vi "Lidar Main V5.2.vi"() -> ()   [LabVIEW 2015]
uses:
  <vilib>/Utility/error.llb/Error Cluster From Error Code.vi
  <vilib>/rvi/errors/niLvFpgaAdjustHostInterfaceError.vi
  Program Files (x86)/National Instruments/LabVIEW 2015/Targets/NI/FPGA/StockFPGA_IntfPrivate/ScriptTemplates/StockFPGA_PlugInRead32.vi
  <vilib>/FPGAPlugInAG/PXIe-7972R/niLvFpga_Abort_PXIe-7972R.vi
  <vilib>/rvi/interface/nirviReadWriteControl/nirviReadWriteControl.xnode
  Controls/FpgaMasterRef Typedef.ctl
  FPGA Bitfiles/LidarMasterV5.1.4.lvbitx
  Controls/FpgaSlaveRef Typedef.ctl
  FPGA Bitfiles/LidarSlaveV5.1.4.lvbitx
  <vilib>/rvi/interface/nirviMethod/nirviMethod.xnode
  <vilib>/rvi/errors/niLvFpgaMergeErrorWithErrorCode.vi
  NiFpgaLv.dll
  <vilib>/FPGAPlugInAG/PXIe-7972R/niLvFpga_Read32_PXIe-7972R.vi
  <vilib>/rvi/interface/nirviReadWriteControl/niFpgaRWControlAccessTimeoutTemplate.vi
  <vilib>/FPGAPlugInAG/PXIe-7972R/niLvFpga_ReadFifo_PXIe-7972R.vi
panel:
  out "RawData":u32[](array[numeric])
  out "error out 2":errorcluster
  out "# elements in queue 2":i32
  out "error out":errorcluster
  in  "SendUDP":bool
  in  "Set VGA Const.":bool
  in  "VGA Val":i16
  out "String":string
  in  "Delay&Close":bool
  in  "SaveToFile":bool
  in  "StartAcq":u16=26 caption="Start Acquisition"
  in  "ActiveSensDeb":u8 caption="Active Sensor"
  in  "SensScanDeb":bool caption="Sensor Scan"
  in  "Active VCSL":u16
  in  "LedScanDebEn":bool=TRUE caption="VCSL Scan"
  in  "Fill VGA":bool
  in  "VGA data":i16[](array[numeric])=[15000, 15000, 15000, 15000, 15000, 15000, 15000, 15000, 15000, 15000, 15000, 15000, 15000, 15000, 15000, 15000, 15000, 15000, 15000, 15000, 15000, 15000, 15000, 15000, 15000, 15000, 15000, 15000, 15000, 15000, 15000, 15000, 15000, 15000, 15000, 15000, 15000, 15000, 15000, 15000, 15000, 15000, 15000, 15000, 15000, 15000, 15000, 15000, 15000, 15000, 15000, 15000, 15000, 15000, 15000, 15000, 15000, 15000, 15000, 15000, 15000, 15000, 15000, 15000, 15000, 15000, 15000, 15000, 15000, 15000, 15000, 15000, 15000, 15000, 15000, 15000, 15000, 15000, 15000, 15000, 15000, 15000, 15000, 15000, 15000, 15000, 15000, 15000, 15000, 15000, 15000, 15000, 15000, 15000, 15000, 15000, 15000, 15000, 15000, 15000]
  in  "PulseEnd":u16=25
  in  "StartPulse":u16=20
  in  "StartES":u16=38
  in  "StopES":u16=44
  in  "SamplingEnable":bool caption="Acquire Frames no Graph"
  in  "AcqMode":bool=TRUE caption="Acq. Mode (T=Raw)"
  in  "SingleFrame":bool caption="Acquire Single Frame"
  out "Samples Amount":i32
  in  "Go":bool caption="Acquire Frames With Graph"
  out "File Error":errorcluster
  in  "CloseFile":bool
  in  "OpenFile":bool
  out "Elements Remaining":u32
  out "Data":i16[][](graph)
  in  "stop":bool
  out "FPGA Error":errorcluster
  # "Acquisition Control"
  # "Timing Control"
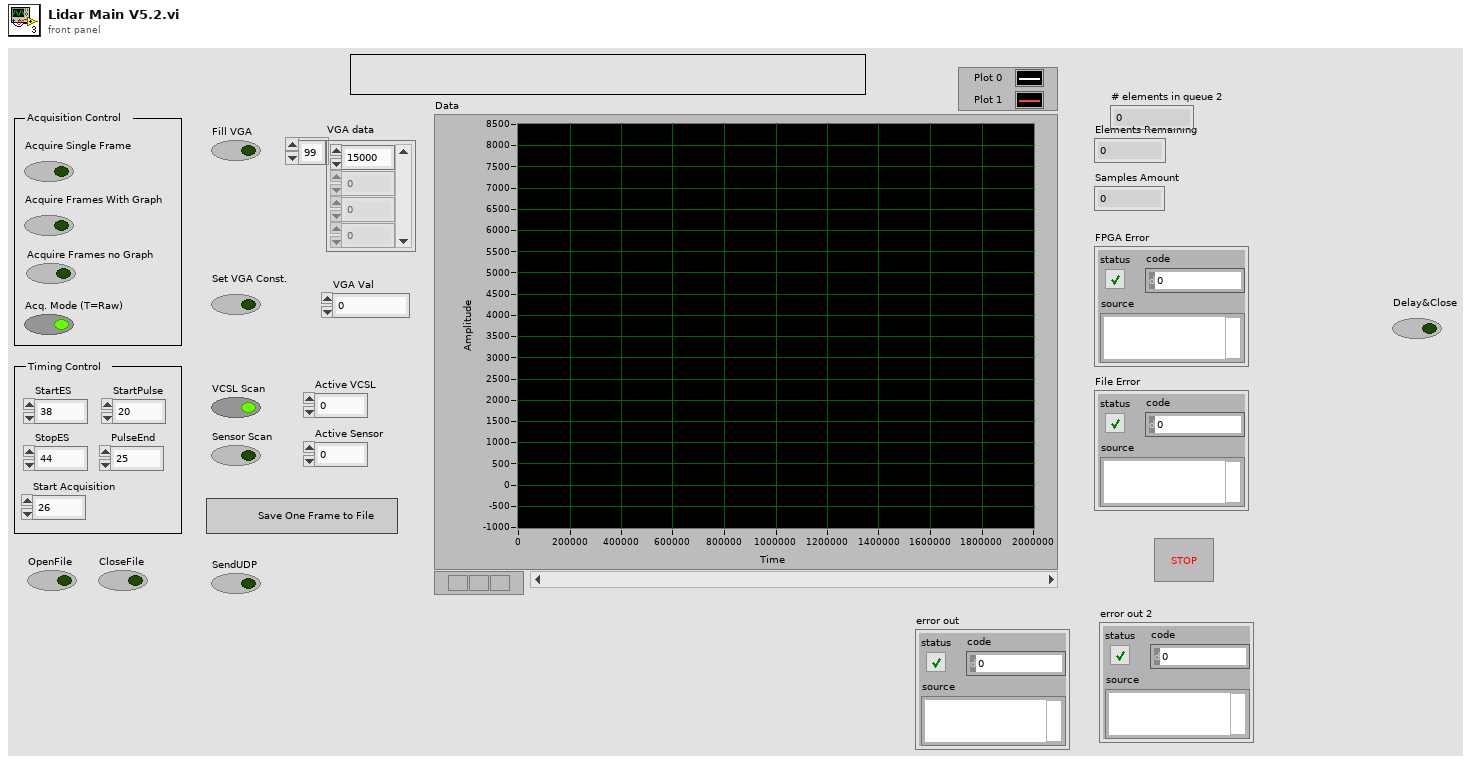
[diagram p1: front panel]
types:
  T1 = enum8{"Internal Clock PLL Off", "Internal Clock PLL On (CLK IN)", "External Clock (CLK IN)", "Internal Clock PLL On (IoModSyncClock)", "Extrernal Clock (IoModSyncClk)"}
  T2 = enum8{"Internal Clock PLL Off", "Internal Clock PLL On (CLK_IN)", "External Clock (CLK_IN)", "Internal Clock PLL On (IoModSyncClk)", "External Clock (IoModSyncClk)"}
  T3 = typedef "FpgaSlaveRef Typedef.ctl" = refnum<k20>
  T4 = typedef "FpgaMasterRef Typedef.ctl" = refnum<k20>
  T5 = enum16{"open", "replace", "create", "open or create", "replace or create", "replace or create with confirmation"}
  T6 = enum16{"big-endian, network order", "native, host order", "little-endian"}
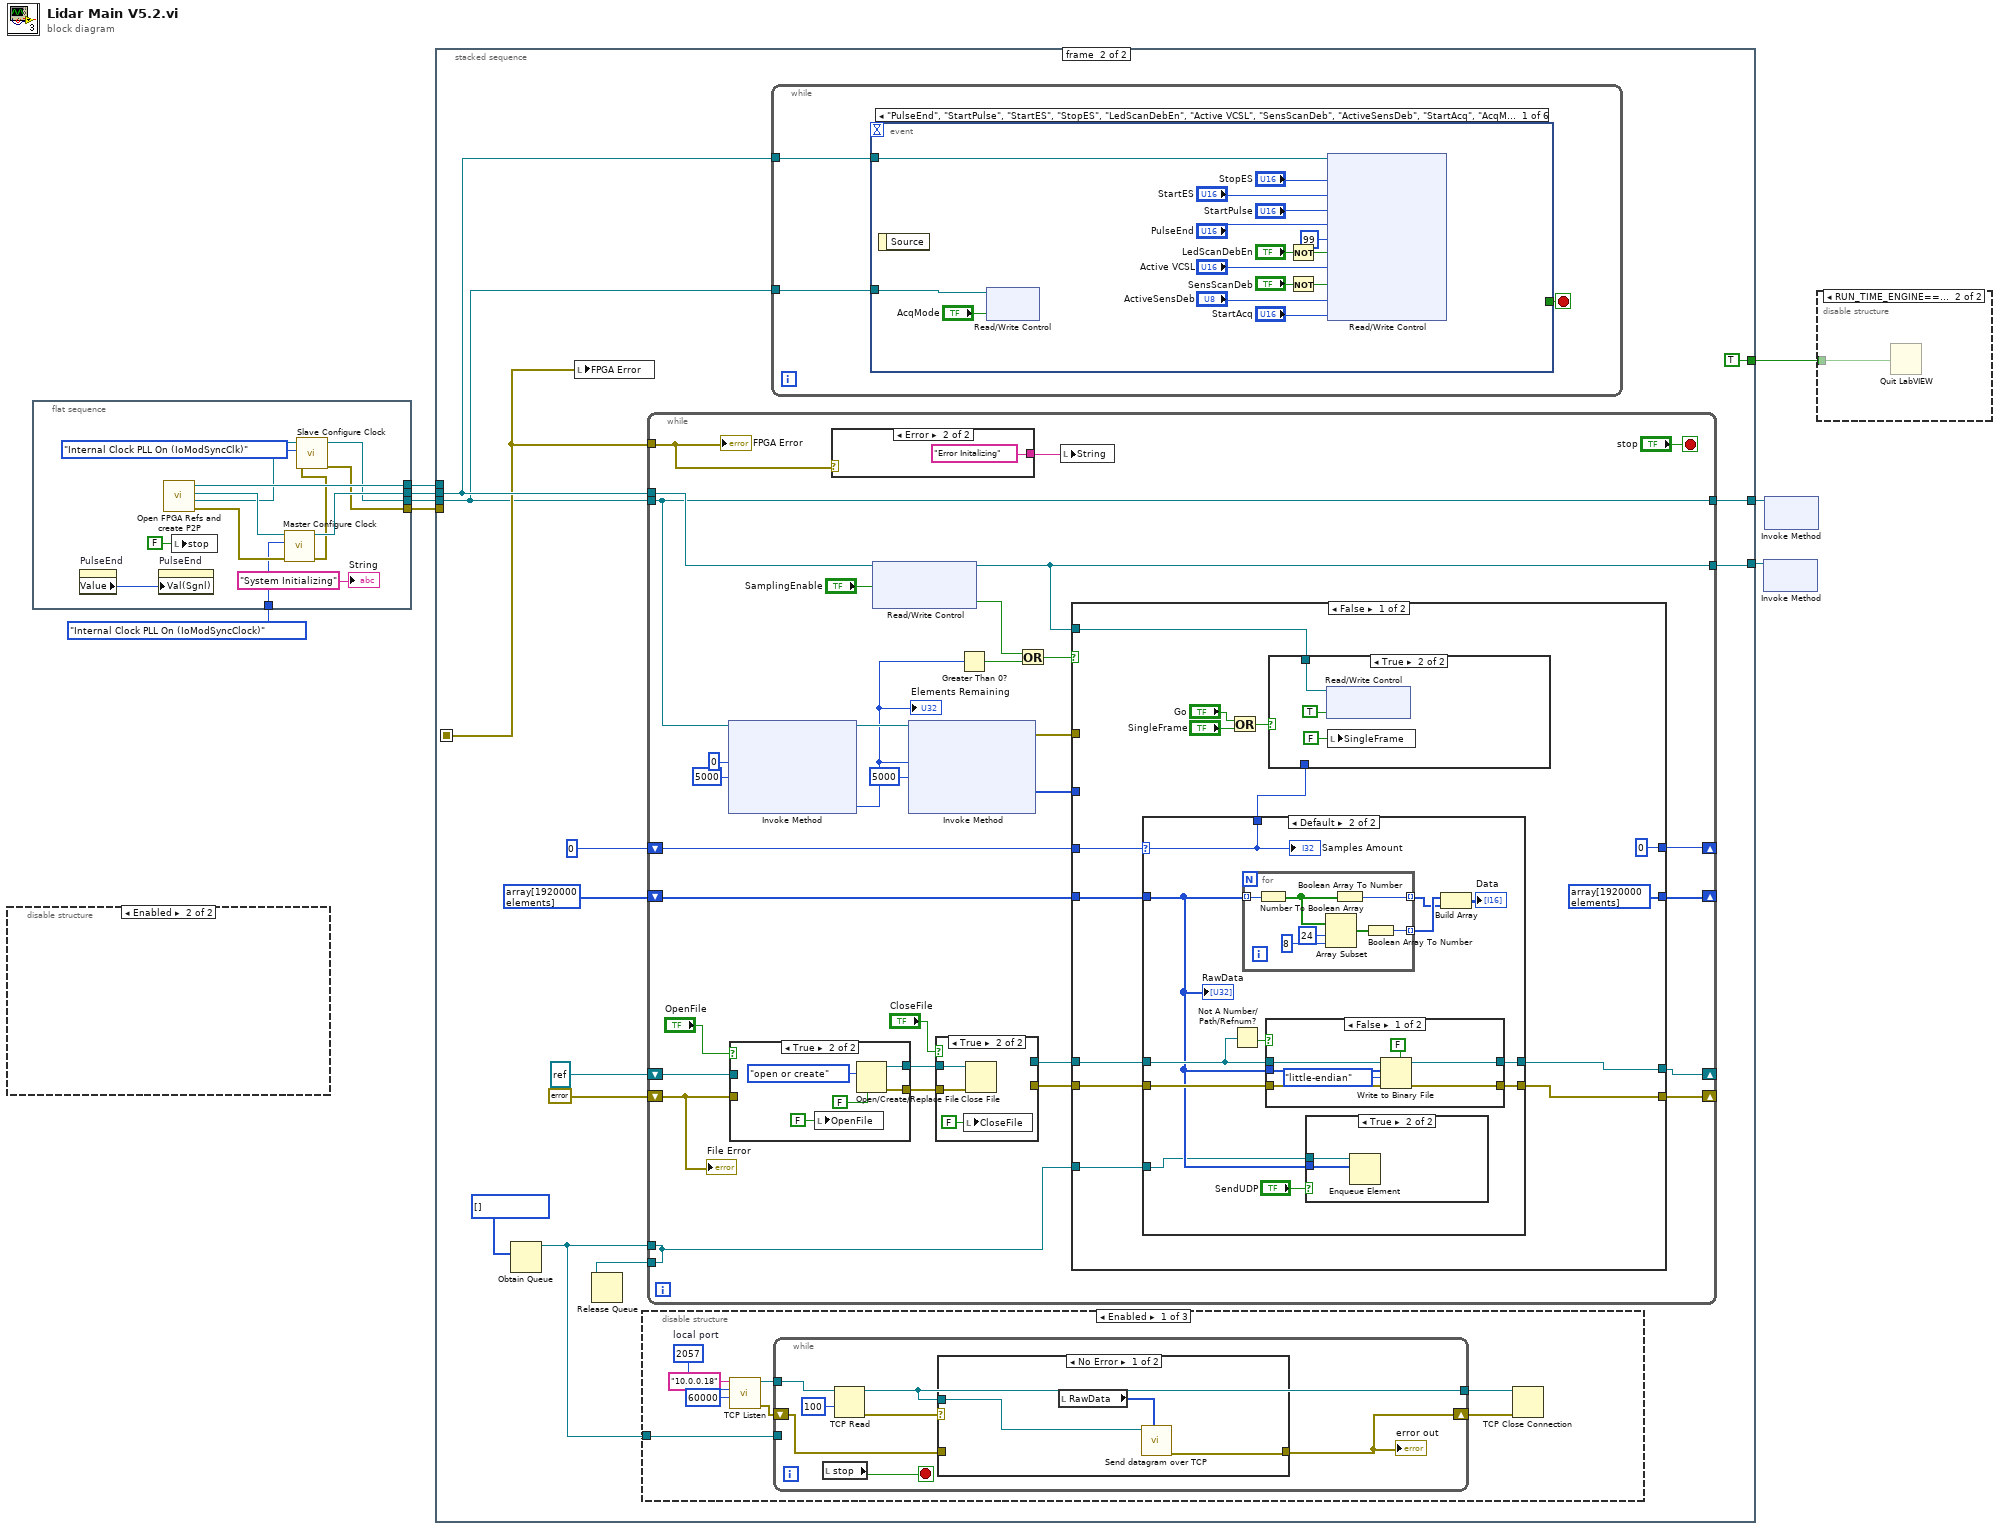
[diagram p0: block diagram]
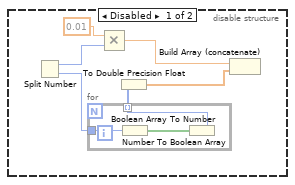
[diagram p3: hidden frame]
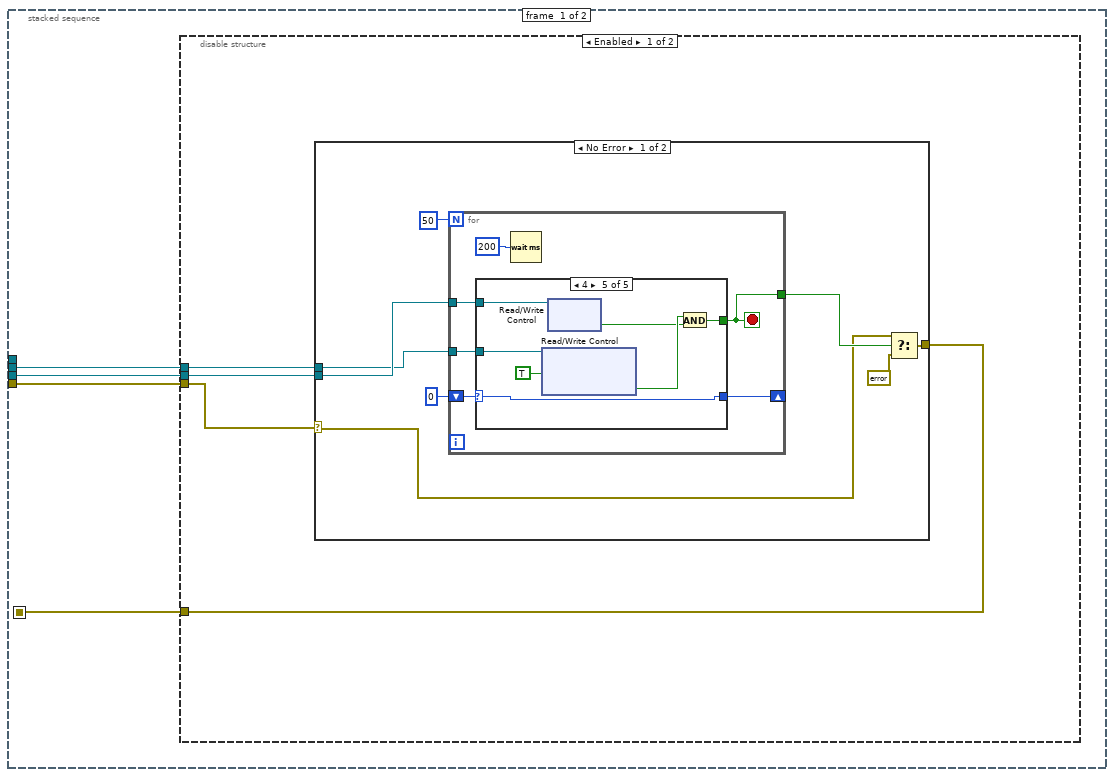
[diagram p4: hidden frame]
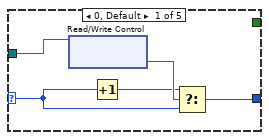
[diagram p5: hidden frame]
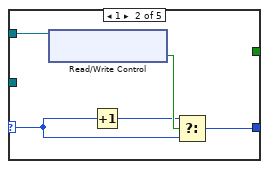
[diagram p6: hidden frame]
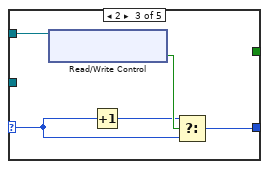
[diagram p7: hidden frame]
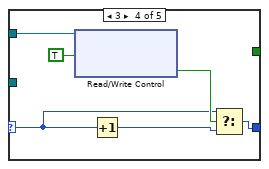
[diagram p8: hidden frame]
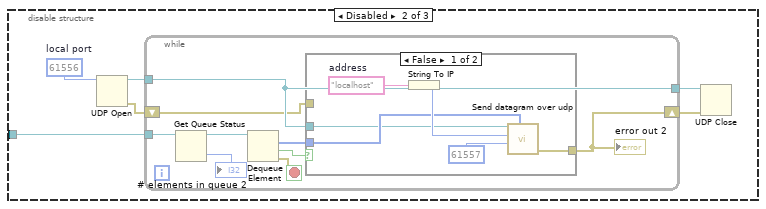
[diagram p12: hidden frame]
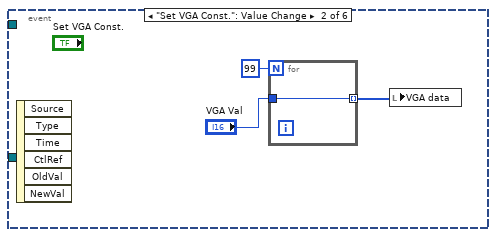
[diagram p15: hidden frame]
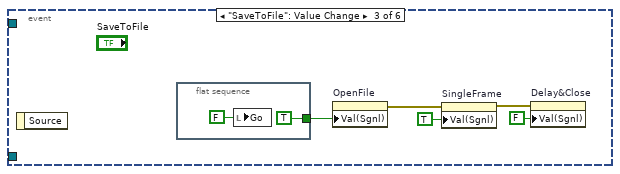
[diagram p16: hidden frame]
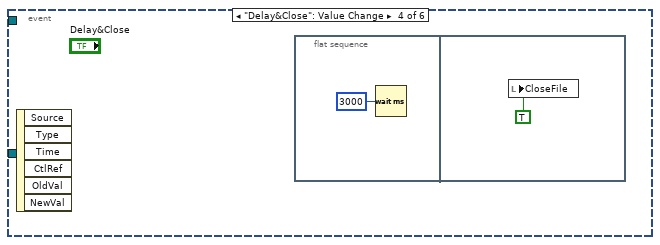
[diagram p17: hidden frame]
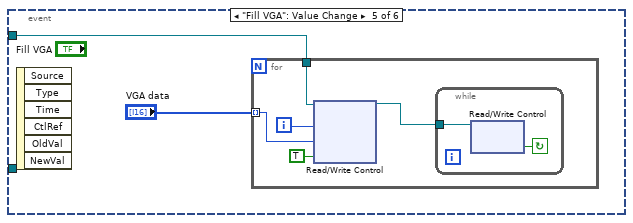
[diagram p18: hidden frame]
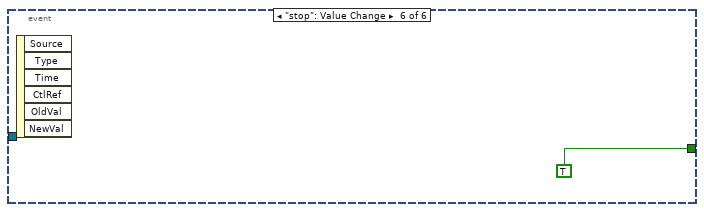
[diagram p19: hidden frame]
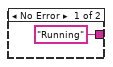
[diagram p20: hidden frame]
diagram:
  n1 = disable-structure shown="Enabled" {
    frame Disabled {
      n2 = Split Number() -> (hi(x)=w10:u16, lo(x)=w14:u16)  [unwired: 1 in]
      n3 = for {
        tunnel: w14 -> [w17]
        tunnel: [w16] -> w11 mode=indexing
        n4 = Number To Boolean Array(number=w17) -> (Boolean array=w15:bool[])
        n5 = Boolean Array To Number(Boolean array=w15) -> (number=w16:i32)
      }
      n6 = Multiply(x=0.01, y=w10) -> (x*y=w9:dbl)
      n7 = To Double Precision Float(number=w11) -> (double precision float=w12:dbl[])
      n8 = Build Array (concatenate)(w9, w12) -> ()  [unwired: 1 out]
    }
    frame Enabled {
    }
  }
  n9 = flat-sequence {
    tunnel: [w30] -> w8
    tunnel: [w20] -> w7
    tunnel: [w22] -> w6
    tunnel: [w26] -> w5
    tunnel: T1."Internal Clock PLL On (IoModSyncClock)" ("Clock Source") -> [w24]
    frame #0 {
      n10 = property on="PulseEnd" class="DigNum (strict)"() -> ("Value"=w28:u16)  [unwired: 2 in, 2 out]
      n11 = property on="PulseEnd" class="DigNum (strict)"("Val(Sgnl)"=w28) -> ()  [unwired: 2 in, 2 out]
      n12 = call "Open FPGA Refs and create P2P.vi"() -> ("error out"=w25:errorcluster, "SlaveRef"=w23:T3, "Master Ref"=w27:T4, "P2P ref"=w30:refnum<k20>)  [unwired: 8 in]
      n13 = local write "stop"(FALSE ("stop")) -> ()
      n14 = call "Master Configure Clock.vi"("error in"=w25, "Clock Source"=w24, "Master Ref"=w27) -> ("error out"=w21:errorcluster, "Master Ref"=w26:T4)  [unwired: 6 in, 1 out]
      n15 = call "Slave Configure Clock.vi"("error in"=w21, "Clock Source"=T2."Internal Clock PLL On (IoModSyncClk)", "SlaveRef"=w23) -> ("error out"=w20:errorcluster, "SlaveRef"=w22:T3)  [unwired: 6 in, 1 out]
      "String" <- "System Initializing" ("String")
    }
  }
  n16 = stacked-sequence {
    seq-local: [w31 _] -> [_ w88]
    tunnel: w8 -> [_ _]
    tunnel: w7 -> [w32 _]
    tunnel: w6 -> [w34 w87]
    tunnel: w5 -> [w33 w91]
    tunnel: [_ w90] -> w4
    tunnel: [_ w89] -> w3
    tunnel: [_ TRUE ("quit? (T)")] -> w1
    frame #0 {
      n17 = disable-structure shown="Enabled" {
        disable-tunnel: w34 -> [w38 _]
        disable-tunnel: w33 -> [w37 _]
        disable-tunnel: w32 -> [w36 w82]
        disable-tunnel: [w35 w82] -> w31
        frame Enabled {
          n18 = case shown="No Error" w36 {
            selector: w36 -> [w41 w81]
            tunnel: w38 -> [w46 _]
            tunnel: w37 -> [w45 _]
            tunnel: [w39 w81] -> w35
            frame No Error {
              n19 = for {
                N: 50 -> [_]
                shift-right: [w49] -> _
                shift-left: u8 0 -> [w52]
                tunnel: w46 -> [w51]
                tunnel: w45 -> [w50]
                tunnel: [w47] -> w42
                stop <- w47 stop-if-true
                n20 = case shown="4" w52 {
                  selector: w52 -> [w54 w60 w65 w69 w74]
                  tunnel: w51 -> [_ w58 w63 w72 w78]
                  tunnel: w50 -> [w57 _ _ _ w79]
                  tunnel: [w55 w61 w66 w73 w74] -> w49
                  tunnel: [_ _ _ _ w75] -> w47
                  frame 0, Default {
                    n21 = xnode "Read/Write Control"("FPGA VI Reference In"=w57) -> ("PLL Locked"=w56:bool)  [unwired: 1 in, 2 out]
                    n22 = Increment(x=w54) -> (x+1=w53:u8)
                    n23 = Select(t=w53, s=w56, f=w54) -> (s? t:f=w55:u8)
                  }
                  frame 1 {
                    n24 = xnode "Read/Write Control"("FPGA VI Reference In"=w58) -> ("Synthesizer Locked"=w62:bool)  [unwired: 1 in, 2 out]
                    n25 = Increment(x=w60) -> (x+1=w59:u8)
                    n26 = Select(t=w59, s=w62, f=w60) -> (s? t:f=w61:u8)
                  }
                  frame 2 {
                    n27 = xnode "Read/Write Control"("FPGA VI Reference In"=w63) -> ("Synthesizer Locked"=w67:bool)  [unwired: 1 in, 2 out]
                    n28 = Increment(x=w65) -> (x+1=w64:u8)
                    n29 = Select(t=w64, s=w67, f=w65) -> (s? t:f=w66:u8)
                  }
                  frame 3 {
                    n30 = xnode "Read/Write Control"("FPGA VI Reference In"=w72, "StartSyncAction"=TRUE) -> ("Trig1"=w70:bool)  [unwired: 1 in, 2 out]
                    n31 = Increment(x=w69) -> (x+1=w68:u8)
                    n32 = Select(t=w69, s=w70, f=w68) -> (s? t:f=w73:u8)
                  }
                  frame 4 {
                    n33 = xnode "Read/Write Control"("FPGA VI Reference In"=w79, "StartSyncLoop"=TRUE ("StartSyncAction")) -> ("Trig1"=w77:bool)  [unwired: 1 in, 2 out]
                    n34 = xnode "Read/Write Control"("FPGA VI Reference In"=w78) -> ("Trig1"=w76:bool)  [unwired: 1 in, 2 out]
                    n35 = And(x=w77, y=w76) -> (x .and. y?=w75:bool)
                  }
                }
                n36 = Wait (ms)(milliseconds to wait=u32 200) -> ()  [unwired: 1 out]
              }
              n37 = Select(t=w41, s=w42, f=errorcluster {"status"=TRUE, "code"=0, "source"="Init Error"}) -> (s? t:f=w39:errorcluster)
            }
            frame Error {
            }
          }
        }
        frame Disabled {
        }
      }
    }
    frame #1 {
      n38 = Obtain Queue(element data type=u32[] []) -> (queue out=w84:refnum<queue>)  [unwired: 4 in, 2 out]
      n39 = local write "FPGA Error"(w88) -> ()
      n40 = disable-structure shown="Enabled" {
        disable-tunnel: w84 -> [w103 w119 _]
        frame Enabled {
          w97 = u16 2057  # local port
          n41 = call <vilib>:"TCP Listen.vi"("timeout ms (wait forever: -1)"=60000 ("timeout ms (60000)"), "port"=w97, "service name"="10.0.0.18" ("address")) -> ("error out"=w100:errorcluster, "connection ID"=w102:refnum<k5>)  [unwired: 4 in, 3 out]
          n42 = while {
            tunnel: w103 -> [_]
            tunnel: w102 -> [w109]
            tunnel: [w108] -> w101
            shift-right: [w110] -> w99
            shift-left: w100 -> [w105]
            stop <- w104 stop-if-true
            n43 = local read "stop"() -> (w104:bool)
            n44 = TCP Read(connection ID=w109, 9:100 ("timeout ms (25000)")) -> (connection ID out=w108:refnum<k5>, error out=w106:errorcluster)  [unwired: 3 in, 1 out]
            n45 = case shown="No Error" w106 {
              tunnel: w108 -> [w113 _]
              tunnel: [w112 w114] -> w110
              tunnel: w105 -> [_ w114]
              frame No Error {
                n46 = local read "RawData"() -> (w111:u32[])
                n47 = call "Send datagram over TCP.vi"("Data"=w111, "connection ID"=w113) -> ("error out"=w112:errorcluster)  [unwired: 9 in]
              }
              frame Error {
              }
            }
            "error out" <- w110
          }
          n48 = TCP Close Connection(connection ID=w101, error in (no error)=w99) -> ()  [unwired: 1 in, 2 out]
        }
        frame Disabled {
          w120 = u16 61556  # local port
          n49 = UDP Open(11:w120) -> (port=w118:refnum<k16>, 0:w116:errorcluster)  [unwired: 4 in, 1 out]
          n50 = while {
            tunnel: w119 -> [w129]
            tunnel: w118 -> [w125]
            tunnel: [w125] -> w117
            shift-right: [w123] -> w115
            shift-left: w116 -> [w124]
            stop <- w126 stop-if-true
            n51 = Get Queue Status(queue=w129) -> (queue out=w122:refnum<queue>, # elements in queue=→"# elements in queue 2":i32)  [unwired: 2 in, 6 out]
            n52 = Dequeue Element(queue=w122) -> (element=w128:u32[], timed out?=w127:bool, error out=w126:errorcluster)  [unwired: 2 in, 1 out]
            n53 = case shown="False" w127 {
              tunnel: w128 -> [w133 _]
              tunnel: w125 -> [w132 _]
              tunnel: w124 -> [_ w136]
              tunnel: [w130 w136] -> w123
              frame False {
                w134 = "localhost"  # address
                n54 = String To IP(1:w134) -> (0:w135:u32)
                n55 = call "Send datagram over udp.vi"("Data"=w133, "port"=u16 61557 ("port or service name"), "Address"=w135, "IDP ref"=w132) -> ("error out"=w130:errorcluster)  [unwired: 7 in]
              }
              frame True {
              }
            }
            "error out 2" <- w123
          }
          n56 = UDP Close(connection ID=w117, 8:w115) -> ()  [unwired: 2 out]
        }
        frame Disabled {
        }
      }
      n57 = while {
        tunnel: w88 -> [w180]
        tunnel: w91 -> [w185]
        tunnel: w87 -> [w181]
        shift-right: [w205] -> _
        shift-left: refnum<file> refnum ("refnum out") -> [w204]
        shift-right: [w202] -> _
        shift-left: errorcluster {"status"=FALSE, "code"=0, "source"=""} ("error out") -> [w201]
        shift-right: [w197] -> _
        shift-left: u32[] array[1920000 elements] -> [w199]
        shift-right: [w198] -> _
        shift-left: 0 -> [w193]
        tunnel: [w182] -> w90
        tunnel: [w181] -> w89
        tunnel: w84 -> [w178]
        tunnel: [w178] -> w83
        stop <- "stop" stop-if-true
        n58 = xnode "Invoke Method"("FPGA VI Reference In"=w181, "Number of Elements"=u32 0, "Timeout (ms)"=5000) -> ("FPGA VI Reference Out"=w208:T3, "Elements Remaining"=w192:u32)  [unwired: 1 in, 2 out]
        "Elements Remaining" <- w192
        n59 = case shown="True" "OpenFile" {
          tunnel: [w218 w223] -> w187
          tunnel: w204 -> [w218 _]
          tunnel: w201 -> [w217 _]
          tunnel: [w217 w222] -> w186
          frame False {
          }
          frame True {
            n60 = local write "OpenFile"(FALSE ("OpenFile")) -> ()
            n61 = Open/Create/Replace File(operation (0:open)=T5."open or create", disable buffering (F)=FALSE) -> (refnum out=w223:refnum<file>, error out=w222:errorcluster)  [unwired: 4 in, 1 out]
          }
        }
        n62 = case shown="Error" w180 {
          tunnel: ["Running" ("String") "Error Initalizing" ("String")] -> w179
          frame No Error {
          }
          frame Error {
          }
        }
        n63 = xnode "Read/Write Control"("FPGA VI Reference In"=w185, "SamplingEnable"="SamplingEnable") -> ("FPGA VI Reference Out"=w182:T4, "SingleFrame"=w183:bool)  [unwired: 1 in, 1 out]
        n64 = xnode "Invoke Method"("FPGA VI Reference In"=w208, "Number of Elements"=w192, "Timeout (ms)"=5000) -> ("error out"=w196:errorcluster, "Data"=w206:u32[])  [unwired: 1 in, 2 out]
        n65 = case shown="True" "CloseFile" {
          tunnel: w187 -> [w213 w216]
          tunnel: [w213 _] -> w203
          tunnel: w186 -> [w212 w215]
          tunnel: [w212 _] -> w200
          frame False {
          }
          frame True {
            n66 = local write "CloseFile"(FALSE ("CloseFile")) -> ()
            n67 = Close File(refnum=w216, error in=w215) -> ()  [unwired: 2 out]
          }
        }
        n68 = Greater Than 0?(x=w192) -> (x > 0?=w191:bool)
        n69 = Or(x=w183, y=w191) -> (x .or. y?=w190:bool)
        n70 = local write "String"(w179) -> ()
        n71 = case shown="False" w190 {
          tunnel: w206 -> [_ w273]
          tunnel: w203 -> [w231 w275]
          tunnel: [w230 w275] -> w205
          tunnel: [w228 w274] -> w202
          tunnel: w200 -> [w229 w274]
          tunnel: w199 -> [w234 w278]
          tunnel: w182 -> [w237 _]
          tunnel: [0 w279] -> w198
          tunnel: w193 -> [w235 w276]
          tunnel: [u32[] array[1920000 elements] w277] -> w197
          tunnel: w196 -> [_ _]
          tunnel: w178 -> [w224 _]
          frame False {
            n72 = case shown="Default" w235 {
              selector: w235 -> [_ w246]
              tunnel: w234 -> [_ w241]
              tunnel: [_ w246] -> w232
              tunnel: w231 -> [w239 w247]
              tunnel: [w239 w251] -> w230
              tunnel: w229 -> [w238 w250]
              tunnel: [w238 w249] -> w228
              tunnel: w224 -> [_ w240]
              frame 0 {
              }
              frame Default {
                n73 = Not A Number/Path/Refnum?(number/path/refnum=w247) -> (NaN/Path/Refnum?=w248:bool)
                n74 = for {
                  tunnel: w241 -> [w256] mode=indexing
                  tunnel: [w254] -> w244 mode=indexing
                  tunnel: [w255] -> w243 mode=indexing
                  n75 = Number To Boolean Array(number=w256) -> (Boolean array=w257:bool[])
                  n76 = Array Subset(array=w257, index=24, length=8) -> (w258:bool[])
                  n77 = Boolean Array To Number(Boolean array=w257) -> (number=w255:i16)
                  n78 = Boolean Array To Number(Boolean array=w258) -> (number=w254:u8)
                }
                n79 = case shown="False" w248 {
                  tunnel: w247 -> [w267 w269]
                  tunnel: [w266 w269] -> w251
                  tunnel: w241 -> [w265 _]
                  tunnel: w250 -> [w264 w268]
                  tunnel: [w263 w268] -> w249
                  frame False {
                    n80 = Write to Binary File(file (use dialog)=w267, data=w265, error in=w264, 5:FALSE ("prepend array or string size? (T)"), 9:T6."little-endian" ("byte order (0:big-endian, network order)")) -> (refnum out=w266:refnum<file>, error out=w263:errorcluster)  [unwired: 1 in, 1 out]
                  }
                  frame True {
                  }
                }
                n81 = case shown="True" "SendUDP" {
                  tunnel: w240 -> [_ w253]
                  tunnel: w241 -> [_ w252]
                  frame False {
                  }
                  frame True {
                    n82 = Enqueue Element(queue=w253, element=w252) -> ()  [unwired: 2 in, 3 out]
                  }
                }
                n83 = Build Array(w244, w243) -> (→"Data":i16[][])
                "Samples Amount" <- w246
                "RawData" <- w241
              }
            }
            n84 = Or(x="Go", y="SingleFrame") -> (x .or. y?=w225:bool)
            n85 = case shown="True" w225 {
              tunnel: w237 -> [_ w272]
              tunnel: w232 -> [_ _]
              frame False {
              }
              frame True {
                n86 = xnode "Read/Write Control"("FPGA VI Reference In"=w272, "SingleFrame"=TRUE) -> ()  [unwired: 1 in, 2 out]
                n87 = local write "SingleFrame"(FALSE ("SingleFrame")) -> ()
              }
            }
          }
          frame True {
            n88 = Array Size(array=w273) -> (size(s)=w280:i32)
            n89 = Add(x=w280, y=w276) -> (x+y=w279:i32)
            n90 = Replace Array Subset(array=w278, new element=w273, index=w276) -> (w277:u32[])
          }
        }
        "File Error" <- w201
        "FPGA Error" <- w180
      }
      n91 = Release Queue(queue=w83) -> ()  [unwired: 2 in, 3 out]
      n92 = while {
        tunnel: w91 -> [w139]
        tunnel: w87 -> [w137]
        stop <- w138 stop-if-true
        n93 = event shown="[0] \"PulseEnd\", \"StartPulse\", \"StartES\", \"StopES\", \"LedScanDebEn\", \"Active VCSL\", \"SensScanDeb\", \"ActiveSensDeb\", \"StartAcq\", \"AcqMode\": Value Change" {
          selector: _ -> [_ _ _ _ _ _]
          dyn-events: _ -> [_ _ _ _ _ _]
          timeout: _ -> [_ _ _ _ _ _]
          tunnel: w139 -> [w154 _ _ _ w168 _]
          tunnel: [_ _ _ _ _ TRUE] -> w138
          tunnel: w137 -> [w145 _ _ _ _ _]
          event "PulseEnd", "StartPulse", "StartES", "StopES", "LedScanDebEn", "Active VCSL", "SensScanDeb", "ActiveSensDeb", "StartAcq", "AcqMode": Value Change {
            n94 = event-data() -> ()  [unwired: 1 in, 1 out]
            n95 = xnode "Read/Write Control"("FPGA VI Reference In"=w145, "Mode"="AcqMode") -> ()  [unwired: 1 in, 2 out]
            n96 = Not(x="LedScanDebEn") -> (.not. x?=w141:bool)
            n97 = Not(x="SensScanDeb") -> (.not. x?=w140:bool)
            n98 = xnode "Read/Write Control"("FPGA VI Reference In"=w154, "StopES"="StopES", "StartES"="StartES", "StartPulse"="StartPulse", "PulseEnd"="PulseEnd", "AiNoOfSamples"=u16 99, "LedScanDebEn"=w141, "ActiveLedIndexDeb"="Active VCSL", "SensScanDeb"=w140, "ActiveSensDeb"="ActiveSensDeb", "StartAcq"="StartAcq") -> ()  [unwired: 1 in, 2 out]
          }
          event "Set VGA Const.": Value Change {
            n99 = event-data() -> ()  [unwired: 1 in, 6 out]
            n100 = for {
              N: 99 -> [_]
              tunnel: [w158] -> w155 mode=indexing
              tunnel: "VGA Val" -> [w158]
            }
            n101 = local write "VGA data"(w155) -> ()
          }
          event "SaveToFile": Value Change {
            n102 = event-data() -> ()  [unwired: 1 in, 1 out]
            n103 = flat-sequence {
              tunnel: [TRUE ("Value (Signaling)")] -> w163
              frame #0 {
                n104 = local write "Go"(FALSE ("Go")) -> ()
              }
            }
            n105 = property on="OpenFile" class="Bool (strict)"("Val(Sgnl)"=w163) -> (error out=w162:errorcluster)  [unwired: 2 in, 1 out]
            n106 = property on="SingleFrame" class="Bool (strict)"(error in=w162, "Val(Sgnl)"=TRUE ("Value (Signaling)")) -> (error out=w160:errorcluster)  [unwired: 1 in, 1 out]
            n107 = property on="Delay&Close" class="Bool (strict)"(error in=w160, "Val(Sgnl)"=FALSE ("Value (Signaling)")) -> ()  [unwired: 1 in, 2 out]
          }
          event "Delay&Close": Value Change {
            n108 = event-data() -> ()  [unwired: 1 in, 6 out]
            n109 = flat-sequence {
              frame #0 {
                n110 = Wait (ms)(milliseconds to wait=u32 3000) -> ()  [unwired: 1 out]
              }
              frame #1 {
                n111 = local write "CloseFile"(TRUE ("CloseFile")) -> ()
              }
            }
          }
          event "Fill VGA": Value Change {
            n112 = event-data() -> ()  [unwired: 1 in, 6 out]
            n113 = for {
              tunnel: w168 -> [w174]
              tunnel: "VGA data" -> [w173] mode=indexing
              i -> [w172]
              n114 = xnode "Read/Write Control"("FPGA VI Reference In"=w174, "VgaAdd"=w172, "VgaData"=w173, "FillVga"=TRUE) -> ("FPGA VI Reference Out"=w171:T4)  [unwired: 1 in, 1 out]
              n115 = while {
                tunnel: w171 -> [w176]
                stop <- w175 continue-if-true
                n116 = xnode "Read/Write Control"("FPGA VI Reference In"=w176) -> ("FillVga"=w175:bool)  [unwired: 1 in, 2 out]
              }
            }
          }
          event "stop": Value Change {
            n117 = event-data() -> ()  [unwired: 1 in, 6 out]
          }
        }
      }
    }
  }
  n118 = xnode "Invoke Method"("FPGA VI Reference In"=w4) -> ()  [unwired: 1 in, 2 out]
  n119 = xnode "Invoke Method"("FPGA VI Reference In"=w3) -> ()  [unwired: 1 in, 2 out]
  n120 = disable-structure shown="RUN_TIME_ENGINE==True" {
    disable-tunnel: w1 -> [_ w281]
    frame condition #0 (active) {
    }
    frame condition #1 {
      n121 = Quit LabVIEW(quit? (T)=w281) -> ()
    }
  }
